vi "运维调试.vi"() -> ()   [LabVIEW 2016]
uses:
  <vilib>/Utility/miscctls.llb/LVPointTypeDef.ctl
  API/AIRMAR WeatherCaster/main.vi
  <vilib>/Utility/config.llb/NI_LVConfig.lvlib
  API/EXO2-Sonde/EXO2-Sonde.lvlib
  API/AIRMAR WeatherCaster/AIRMAR WeatherCaster.lvlib
  API/Section_monitoring_system/function/main/main.lvlib
panel:
  in  "运维调试菜单":T1(xcontrol)
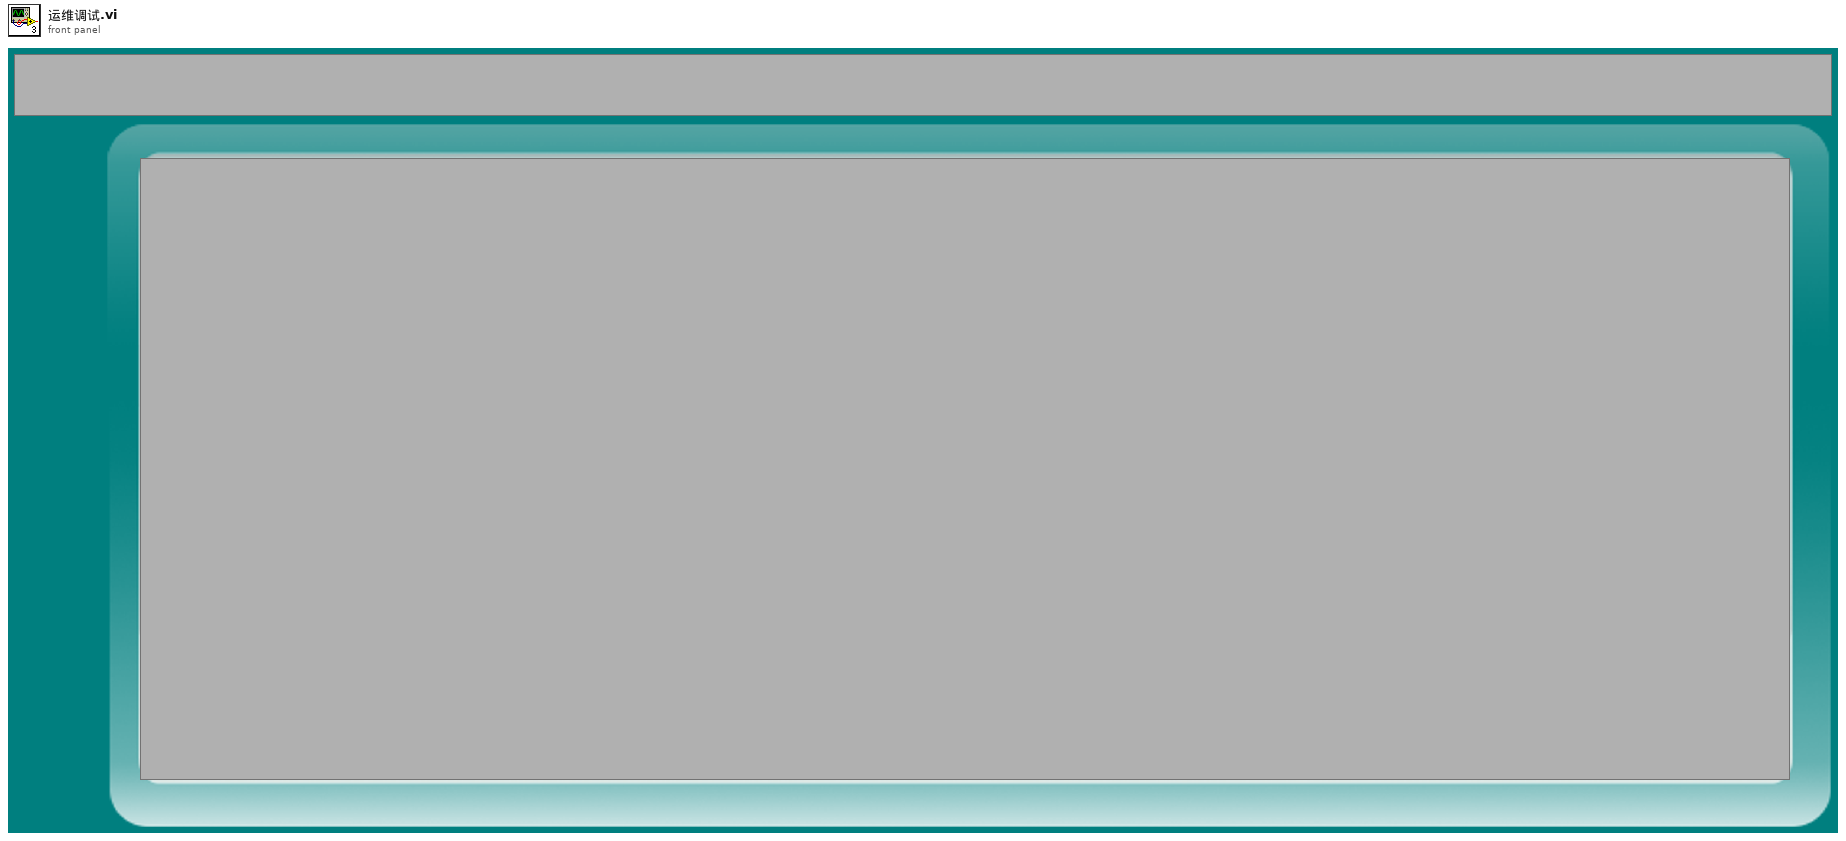
[diagram p1: front panel]
types:
  T1 = enum16{"采配水", "氨氮", "总磷", "总氮", "高锰酸盐指数", "化学需氧量", "多参数", "加标回收", "气象", "EXO2", "剖面系统"}
  T2 = typedef "LVPointTypeDef.ctl" = cluster{"Horizontal":i16, "Vertical":i16}
  T3 = typedef "NI_LVConfig.lvlib/Config Data RefNum.ctl" = refnum<k1>
  T4 = cluster{"采配水":bool, "氨氮":bool, "总磷":bool, "总氮":bool, "高锰酸盐指数":bool, "化学需氧量":bool, "多参数":bool, "加标回收":bool, "气象":bool, "多参数版本":enum16{"集成", "原位"}, "EXO2 Sonde":bool, "剖面系统":bool, "CODMn版本":enum16{"PLC版", "单片机版"}}
  T5 = cluster{"采配水":bool, "氨氮":bool, "总磷":bool, "总氮":bool, "高锰酸盐指数":bool, "化学需氧量":bool, "多参数":bool, "加标回收":bool, "气象":bool, "EXO2 Sonde":bool, "剖面系统":bool}
  T6 = enum32{"Bad", "Idle", "Run top level", "Running"}
  T7 = cluster{"环境动力":string, "氨氮":string, "总磷":string, "总氮":string, "高锰酸盐指数":string, "化学需氧量":string, "多参数":string, "加标回收":string, "气象":string, "EXO2":string, "剖面系统":string}
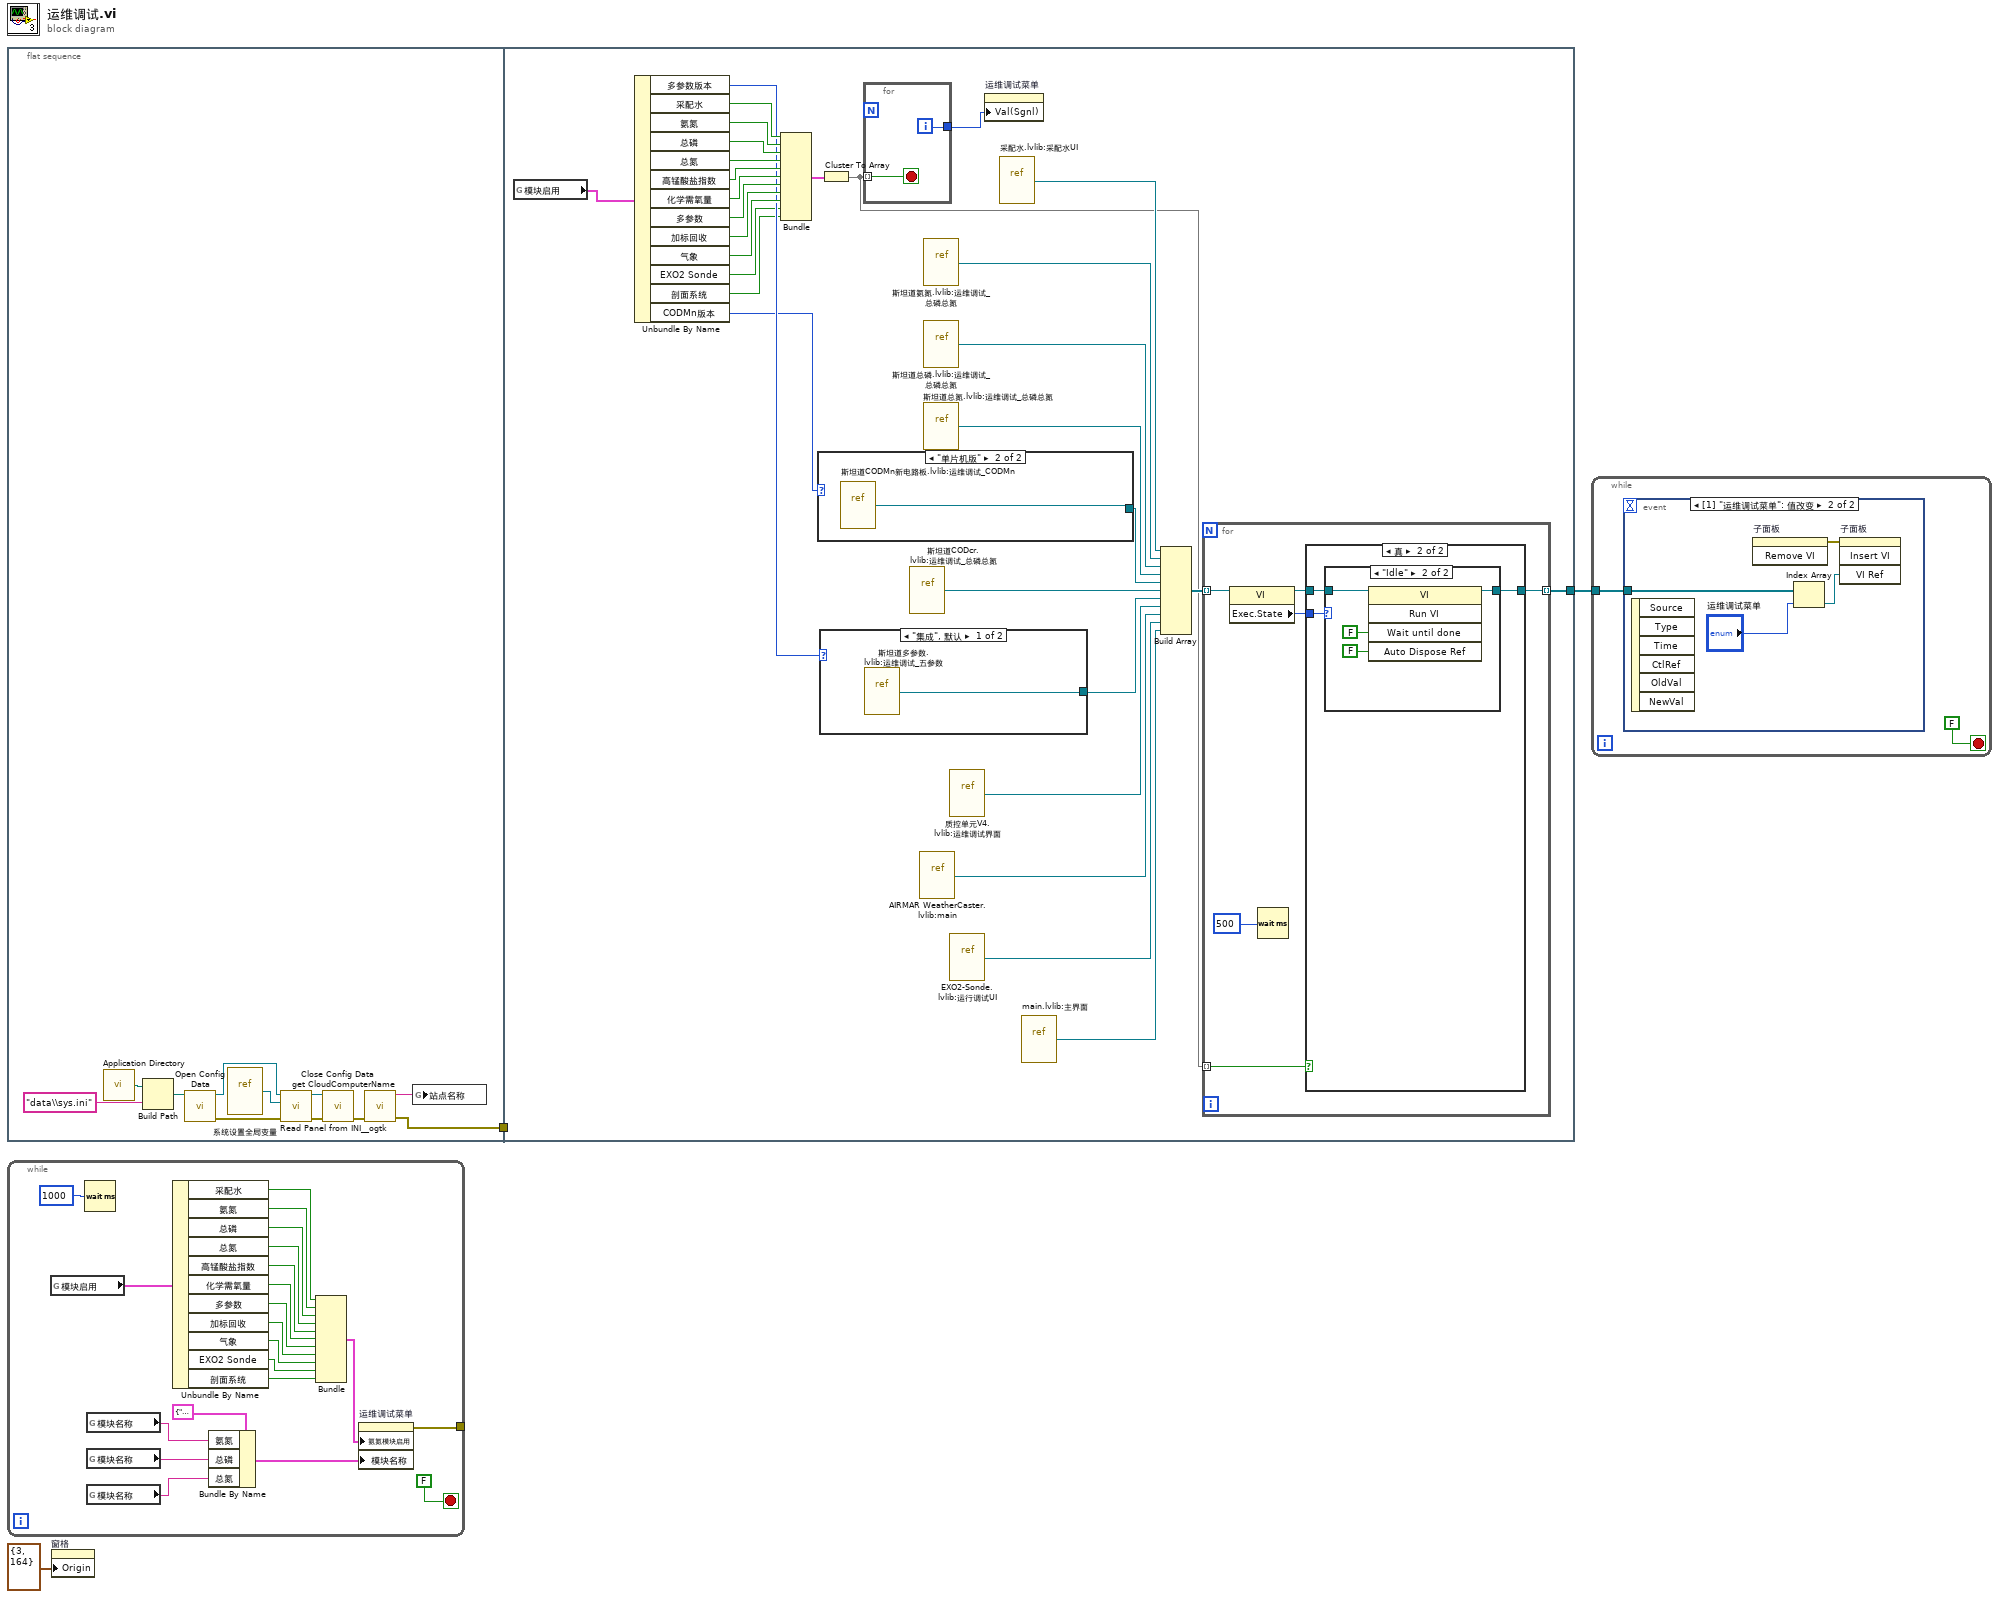
[diagram p0: block diagram]
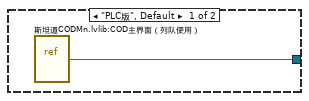
[diagram p2: hidden frame]
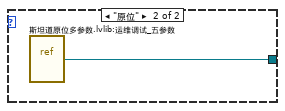
[diagram p3: hidden frame]
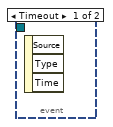
[diagram p6: hidden frame]
diagram:
  n1 = flat-sequence {
    tunnel: [w5] -> w1
    tunnel: w1 -> [_]
    tunnel: [w44] -> w2
    frame #0 {
      n2 = call <vilib>:"Application Directory.vi"() -> ("Application Directory"=w7:path)
      n3 = Build Path(base path=w7, name or relative path="data\\sys.ini" ("名称或相对路径")) -> (appended path=w9:path)
      n4 = call <vilib>:"Open Config Data.vi"("configuration file path"=w9) -> ("error out"=w13:errorcluster, "refnum"=w10:T3)  [unwired: 8 in, 1 out]
      n5 = vi-ref "系统设置全局变量.vi"() -> (w11:refnum<vi>)
      n6 = call <userlib>:"Read Panel from INI__ogtk.vi"("error in (no error)"=w13, "VI ref"=w11, "refnum"=w10) -> ("error out"=w14:errorcluster, "refnum out"=w12:T3)  [unwired: 7 in]
      n7 = call <vilib>:"Close Config Data.vi"("error in (no error)"=w14, "refnum"=w12) -> ("error out"=w6:errorcluster)  [unwired: 8 in, 1 out]
      n8 = call "get CloudComputerName.vi"("error in (no error)"=w6) -> ("error out"=w5:errorcluster, "String/Binary data"=w4:string)  [unwired: 9 in]
      n9 = global write "系统设置全局变量.vi" "站点名称"(w4) -> ()
    }
    frame #1 {
      n10 = global read "系统设置全局变量.vi" "模块启用"() -> (w33:T4)
      n11 = Unbundle By Name(w33) -> ("多参数版本"=w22:enum16{"集成", "原位"}, "采配水"=w32:bool, "氨氮"=w31:bool, "总磷"=w30:bool, "总氮"=w29:bool, "高锰酸盐指数"=w28:bool, "化学需氧量"=w27:bool, "多参数"=w26:bool, "加标回收"=w25:bool, "气象"=w24:bool, "EXO2 Sonde"=w20:bool, "剖面系统"=w16:bool, "CODMn版本"=w15:enum16{"PLC版", "单片机版"})
      n12 = Bundle("采配水"=w32, "氨氮"=w31, "总磷"=w30, "总氮"=w29, "高锰酸盐指数"=w28, "化学需氧量"=w27, "多参数"=w26, "加标回收"=w25, "气象"=w24, "EXO2 Sonde"=w20, "剖面系统"=w16) -> (w23:T5)  [unwired: 1 in]
      n13 = case shown="\"单片机版\"" w15 {
        tunnel: [w45 w46] -> w38
        frame "PLC版", Default {
          n14 = vi-ref "斯坦道CODMn.lvlib:COD主界面（列队使用）.vi"() -> (w45:refnum<vi>)
        }
        frame "单片机版" {
          n15 = vi-ref "斯坦道CODMn新电路板.lvlib:运维调试_CODMn.vi"() -> (w46:refnum<vi>)
        }
      }
      n16 = case shown="\"集成\", 默认" w22 {
        tunnel: [w49 w50] -> w37
        frame "集成", Default {
          n17 = vi-ref "斯坦道多参数.lvlib:运维调试_五参数.vi"() -> (w49:refnum<vi>)
        }
        frame "原位" {
          n18 = vi-ref "斯坦道原位多参数.lvlib:运维调试_五参数.vi"() -> (w50:refnum<vi>)
        }
      }
      n19 = Cluster To Array(cluster=w23) -> (array=w19:bool[])
      n20 = for {
        tunnel: w19 -> [w48] mode=indexing
        tunnel: [w47] -> w18
        i -> [w47]
        stop <- w48 stop-if-true
      }
      n21 = vi-ref "斯坦道CODcr.lvlib:运维调试_总磷总氮.vi"() -> (w34:refnum<vi>)
      n22 = vi-ref "AIRMAR WeatherCaster.lvlib:main.vi"() -> (w35:refnum<vi>)
      n23 = vi-ref "斯坦道氨氮.lvlib:运维调试_总磷总氮.vi"() -> (w42:refnum<vi>)
      n24 = vi-ref "斯坦道总磷.lvlib:运维调试_总磷总氮.vi"() -> (w40:refnum<vi>)
      n25 = vi-ref "斯坦道总氮.lvlib:运维调试_总磷总氮.vi"() -> (w39:refnum<vi>)
      n26 = vi-ref "质控单元V4.lvlib:运维调试界面.vi"() -> (w36:refnum<vi>)
      n27 = vi-ref "EXO2-Sonde.lvlib:运行调试UI.vi"() -> (w21:refnum<vi>)
      n28 = property on="运维调试菜单" class="运维调试菜单 (严格)"("Val(Sgnl)"=w18) -> ()  [unwired: 2 in, 2 out]
      n29 = vi-ref "采配水.lvlib:采配水UI.vi"() -> (w41:refnum<vi>)
      n30 = vi-ref "main.lvlib:主界面.vi"() -> (w17:refnum<vi>)
      n31 = Build Array(w41, w42, w40, w39, w38, w34, w37, w36, w35, w21, w17) -> (w43:refnum<vi>[])
      n32 = for {
        tunnel: w43 -> [w56] mode=indexing
        tunnel: [w55] -> w44 mode=indexing
        tunnel: w19 -> [w52] mode=indexing
        n33 = property class="VI"(reference=w56) -> (reference out=w53:refnum<vi>, "Exec.State"=w54:T6)  [unwired: 1 in, 1 out]
        n34 = Wait (ms)(milliseconds to wait=u32 500 ("等待时间（毫秒）")) -> ()  [unwired: 1 out]
        n35 = case shown="真" w52 {
          tunnel: [w57 w60] -> w55
          tunnel: w54 -> [_ w59]
          tunnel: w53 -> [w57 w58]
          frame False {
          }
          frame True {
            n36 = case shown="\"Idle\"" w59 {
              tunnel: w58 -> [w61 w63]
              tunnel: [w61 w62] -> w60
              frame "Bad", Default {
              }
              frame "Idle" {
                n37 = invoke class="VI" method="Run VI"(reference=w63, "Wait until done"=FALSE ("结束前等待"), "Auto Dispose Ref"=FALSE ("自动销毁引用")) -> (reference out=w62:refnum<vi>)  [unwired: 2 in, 4 out]
              }
            }
          }
        }
      }
    }
  }
  n38 = while {
    tunnel: [w81] -> _
    stop <- FALSE stop-if-true
    n39 = global read "系统设置全局变量.vi" "模块启用"() -> (w79:T4)
    n40 = Wait (ms)(milliseconds to wait=u32 1000 ("等待时间（毫秒）")) -> ()  [unwired: 1 out]
    n41 = global read "VAR总磷总氮全局变量.vi" "模块名称"() -> (w82:string)
    n42 = global read "VAR总磷总氮全局变量.vi" "模块名称"() -> (w84:string)
    n43 = global read "VAR总磷总氮全局变量.vi" "模块名称"() -> (w83:string)
    n44 = Unbundle By Name(w79) -> ("采配水"=w78:bool, "氨氮"=w77:bool, "总磷"=w76:bool, "总氮"=w75:bool, "高锰酸盐指数"=w74:bool, "化学需氧量"=w73:bool, "多参数"=w72:bool, "加标回收"=w71:bool, "气象"=w70:bool, "EXO2 Sonde"=w68:bool, "剖面系统"=w67:bool)
    n45 = Bundle By Name(cluster=T7 {"环境动力"="采配水", "氨氮"="氨氮", "总磷"="总磷", "总氮"="总氮", "高锰酸盐指数"="CODMn", "化学需氧量"="CODcr", "多参数"="多参数", "加标回收"="加标回收", "气象"="气象", "EXO2"="EXO2", "剖面系统"="剖面系统"} ("Value"), "氨氮"=w82, "总磷"=w84, "总氮"=w83) -> (w66:T7)
    n46 = Bundle("采配水"=w78, "氨氮"=w77, "总磷"=w76, "总氮"=w75, "高锰酸盐指数"=w74, "化学需氧量"=w73, "多参数"=w72, "加标回收"=w71, "气象"=w70, "EXO2 Sonde"=w68, "剖面系统"=w67) -> (w69:T5)  [unwired: 1 in]
    n47 = property on="运维调试菜单" class="运维调试菜单 (严格)"("氨氮模块启用"=w69, "模块名称"=w66) -> (error out=w81:errorcluster)  [unwired: 2 in, 1 out]
  }
  n48 = property on="窗格" class="Pane"("Origin"=T2 {"Horizontal"=3, "Vertical"=164} ("原点")) -> ()  [unwired: 2 in, 2 out]
  n49 = while {
    tunnel: w2 -> [w87]
    stop <- FALSE stop-if-true
    n50 = event shown="[1] \"运维调试菜单\": 值改变" {
      selector: _ -> [_ _]
      dyn-events: _ -> [_ _]
      timeout: _ -> [_ _]
      tunnel: w87 -> [_ w91]
      event Timeout {
        n51 = event-data() -> ()  [unwired: 1 in, 3 out]
      }
      event "运维调试菜单": Value Change {
        n52 = event-data() -> ()  [unwired: 1 in, 6 out]
        n53 = invoke on="子面板" class="SubPnl" method="Remove VI"() -> (error out=w92:errorcluster)  [unwired: 3 in, 2 out]
        n54 = Index Array(array=w91, index="运维调试菜单") -> (element=w90:refnum<vi>)
        n55 = invoke on="子面板" class="SubPnl" method="Insert VI"(error in=w92, "VI Ref"=w90) -> ()  [unwired: 2 in, 4 out]
      }
    }
  }
